vi "FRCts20_Backend_Division_PUT.vi"(6 "Message Attributes":T4, 8 "error in (no error)":errorcluster, 10 "Data":string, 11 "Engine_Refnums":T1) -> (0 "error out":errorcluster)   [LabVIEW 2014]
doc: "Adds many teams to a selected division. Called by the division/team api, and expects a division location and an array of team numbers."
uses:
  Dependencies/Keyed Array/KeyedArray.ctl
  FRCts20_Backend_EngineRefnums.ctl
  INI_Accessor/FRCts20_Backend_INI Controller.lvclass
  Dependencies/AMC/_SubVIs/TypeDefs/Message Queue.ctl
  Dependencies/AMC/_SubVIs/TypeDefs/Message.ctl
  <vilib>/addons/database/Connection.llb/Conn ObjectReference.ctl
  FRCts20_Backend_FGVOperation.ctl
  FRCts20_Backend_API/FRCts20_Backend_API_Division.ctl
  FRCts20_Backend_API/FRCts20_Backend_API_SW.ctl
  FRCts20_Backend_API/FRCts20_Backend_API_Status.ctl
  FRCts20_Backend_Engine.lvlib
  FRCts20_Backend_API/FRCts20_Backend_API.lvlib
  Dependencies/Keyed Array/Tools_KeyedArray.lvlib
  Dependencies/AMC/AMC.lvlib
  <vilib>/addons/database/NI_Database_API.lvlib
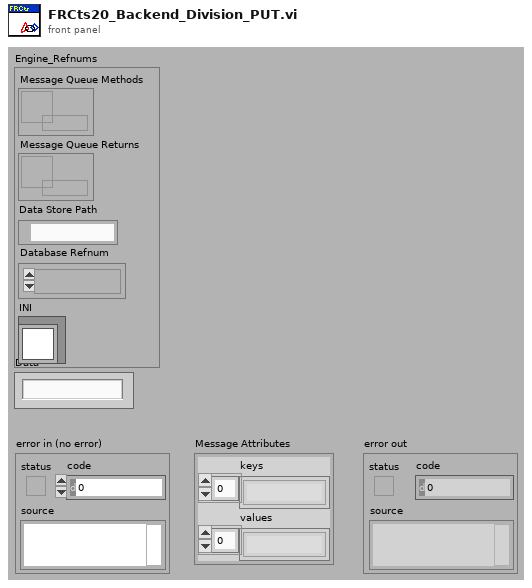
[diagram p1: front panel]
types:
  T1 = typedef "FRCts20_Backend_Engine.lvlib/FRCts20_Backend_EngineRefnums.ctl" = cluster{"Message Queue Methods":T2, "Message Queue Returns":T2, "Data Store Path":path, "Database Refnum":T3, "INI":refnum<class "FRCts20_Backend_INI Controller.lvclass">}
  T2 = typedef "AMC.lvlib/Message Queue.ctl" = refnum<queue>
  T3 = typedef "NI_Database_API.lvlib/Conn ObjectReference.ctl" = refnum<k1>
  T4 = typedef "Tools_KeyedArray.lvlib/KeyedArray.ctl" = cluster{"keys":string[], "values":string[]}
  T5 = typedef "FRCts20_Backend_API.lvlib/FRCts20_Backend_API_Division.ctl" = cluster{"Location":string, "Team":u32[], "APIReturn":string, "RootCmd":enum16{"Issues", "Software", "All"}, "SWType":T6, "Status":T7, "Competition":string}
  T6 = typedef "FRCts20_Backend_API.lvlib/FRCts20_Backend_API_SW.ctl" = string
  T7 = typedef "FRCts20_Backend_API.lvlib/FRCts20_Backend_API_Status.ctl" = enum16{"Open", "In Work", "Closed"}
  T8 = typedef "FRCts20_Backend_Engine.lvlib/FRCts20_Backend_FGVOperation.ctl" = enum16{"Initialize", "EnqueueMessage", "EnqueueDataReturn", "FlushMessage", "FlushDataReturn"}
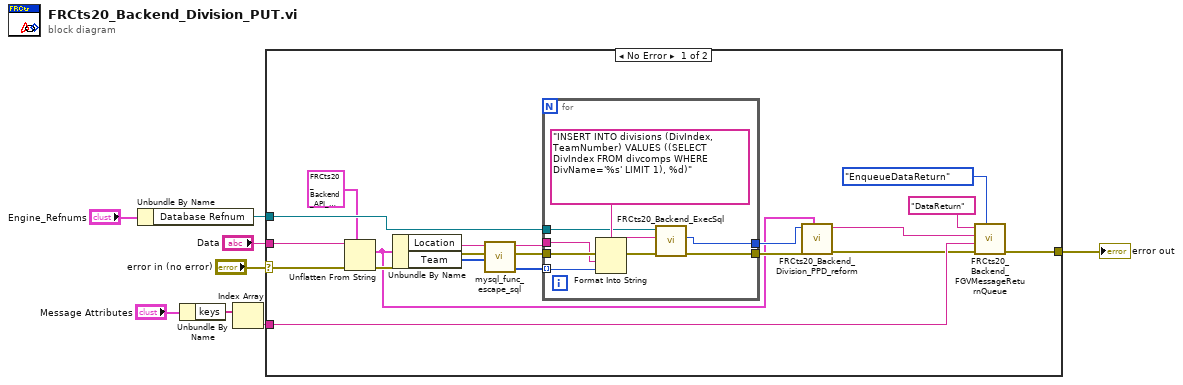
[diagram p0: block diagram]
diagram:
  n1 = Unbundle By Name("Engine_Refnums") -> ("Database Refnum"=w5:T3)
  n2 = Unbundle By Name("Message Attributes") -> ("keys"=w2:string[])
  n3 = Index Array(array=w2) -> (element=w1:string)  [unwired: 1 in]
  n4 = case shown="No Error" "error in (no error)" {
    selector: "error in (no error)" -> [w23 w36]
    tunnel: [w26 w36] -> w7
    tunnel: w5 -> [w19 _]
    tunnel: "Data" -> [w24 _]
    tunnel: w1 -> [w25 _]
    frame No Error {
      n5 = Unflatten From String(type=T5 {"Location"="", "Team"=[], "APIReturn"="", "RootCmd"=enum."Issues", "SWType"="", "Status"=enum."Open", "Competition"=""} ("Division"), binary string=w24, error in (no error)=w23) -> (value=w11:T5, error out=w22:errorcluster)  [unwired: 2 in, 1 out]
      n6 = Unbundle By Name(w11) -> ("Location"=w14:string, "Team"=w17:u32[])
      n7 = call "mysql_func_escape_sql.vi"("error in (no error)"=w22, "sqlin"=w14) -> ("error out"=w16:errorcluster, "escaped"=w15:string)  [unwired: 8 in]
      n8 = for {
        tunnel: w19 -> [w31]
        tunnel: [w27] -> w12
        tunnel: w17 -> [w33] mode=indexing
        tunnel: w15 -> [w32]
        tunnel: w16 -> [w35]
        tunnel: [w28] -> w13
        n9 = Format Into String(format string="INSERT INTO divisions (DivIndex, TeamNumber) VALUES ((SELECT DivIndex FROM divcomps WHERE DivName='%s' LIMIT 1), %d)", error in=w35, w32, w33) -> (resulting string=w30:string, error out=w29:errorcluster)  [unwired: 1 in]
        n10 = call "FRCts20_Backend_ExecSql.vi"("error in (no error)"=w29, "format string"=w30, "Refnum in"=w31) -> ("error out"=w28:errorcluster, "rows affected"=w27:i32)  [unwired: 6 in, 1 out]
      }
      n11 = call "FRCts20_Backend_Division_PPD_reform.vi"("Division"=w11, "error in (no error)"=w13, "rows affected"=w12) -> ("error out"=w10:errorcluster, "data string"=w9:string)  [unwired: 7 in]
      n12 = call "FRCts20_Backend_FGVMessageReturnQueue.vi"("Operation"=FRCts20_Backend_FGVOperation."EnqueueDataReturn", "error in (no error)"=w10, "Key"=w25, "Message Value"=w9, "Message Name"="DataReturn") -> ("error out"=w26:errorcluster)  [unwired: 5 in, 1 out]
    }
    frame Error {
    }
  }
  "error out" <- w7
